vi "Initialize.vi"(8 "error in (no error)":errorcluster {"code" format="Error %.0f"}) -> (0 "error out":errorcluster {"code" format="Error %.0f"}, 2 "UI Events":T1, 3 "Progress Bar UI Out":refnum<class "Progress Bar UI.lvclass">)   [LabVIEW 2023, in "Progress Bar UI.lvclass"]
uses:
  Progress Bar UI.lvclass
  Progress Bar UI.lvclass/Progress Bar UI.ctl
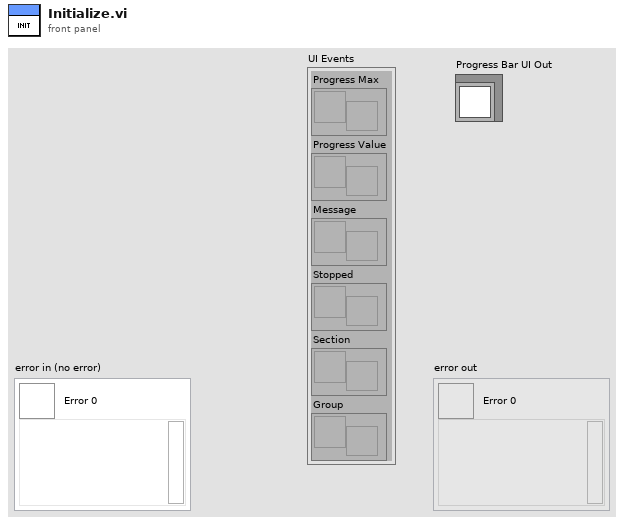
[diagram p1: front panel]
types:
  T1 = cluster{"Progress Max":refnum<user-event>, "Progress Value":refnum<user-event>, "Message":refnum<user-event>, "Stopped":refnum<user-event>, "Section":refnum<user-event>, "Group":refnum<user-event>}
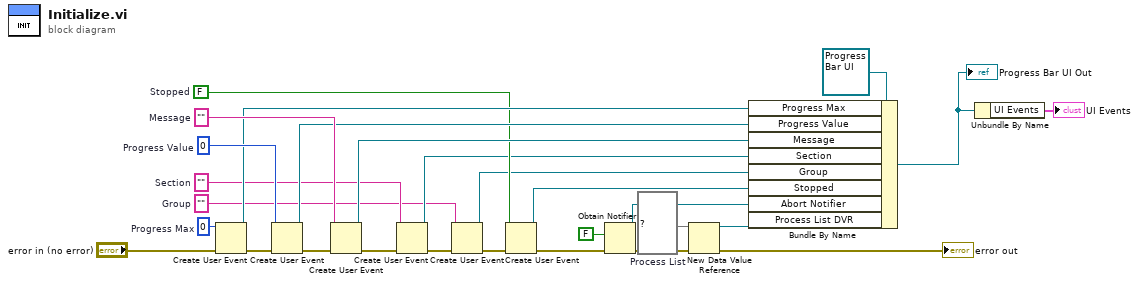
[diagram p0: block diagram]
diagram:
  w4 = set{string} {}  # Process List
  w7 = ""  # Group
  w9 = ""  # Section
  w13 = FALSE  # Stopped
  w22 = ""  # Message
  w25 = 0  # Progress Value
  w26 = 0  # Progress Max
  n1 = Create User Event(user event datatype=w26, error in="error in (no error)") -> (user event=w16:refnum<user-event>, error out=w24:errorcluster)
  n2 = Create User Event(user event datatype=w25, error in=w24) -> (user event=w17:refnum<user-event>, error out=w23:errorcluster)
  n3 = Create User Event(user event datatype=w22, error in=w23) -> (user event=w18:refnum<user-event>, error out=w11:errorcluster)
  n4 = Create User Event(user event datatype=w9, error in=w11) -> (user event=w8:refnum<user-event>, error out=w10:errorcluster)
  n5 = Create User Event(user event datatype=w7) -> (user event=w6:refnum<user-event>)  [unwired: 1 in, 1 out]
  n6 = Create User Event(user event datatype=w13, error in=w10) -> (user event=w12:refnum<user-event>, error out=w14:errorcluster)
  n7 = Obtain Notifier(notification data type=FALSE, error in (no error)=w14) -> (notifier out=w19:refnum<notifier>, error out=w3:errorcluster)  [unwired: 2 in, 1 out]
  n8 = New Data Value Reference(data value=w4, error in=w3) -> (data value reference=w2:refnum<data-value>, error out=→"error out":errorcluster)
  n9 = Bundle By Name(cluster=refnum<class "Progress Bar UI.lvclass"> refnum ("Progress Bar UI out"), "Progress Max"=w16, "Progress Value"=w17, "Message"=w18, "Section"=w8, "Group"=w6, "Stopped"=w12, "Abort Notifier"=w19, "Process List DVR"=w2) -> (w15:refnum<class "Progress Bar UI.lvclass">)
  "Progress Bar UI Out" <- w15
  n10 = Unbundle By Name(w15) -> ("UI Events"=→"UI Events":T1)
